vi "AtSpectrograph_logEvent_STRING.vi"(8 "error in (no error)":errorcluster, 11 "logevent_STRING_Ctl":T1) -> (0 "error out":errorcluster, 2 "function return":i32, 3 "logevent_STRING_Ctl out":T1)   [LabVIEW 2016, in "SALLV_AtSpectrograph.lvlib"]
doc: "int AtSpectrograph_shm_logEvent_STRINGLV(AtSpectrograph_logevent_STRINGLV *logevent_STRING_Ctl );"
uses:
  SALLV_AtSpectrograph.lvlib
  DataTypes/logevent_STRING.ctl
  SALLV_AtSpectrograph.so
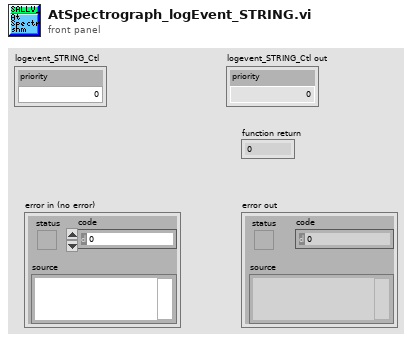
[diagram p1: front panel]
types:
  T1 = typedef "SALLV_AtSpectrograph.lvlib/logevent_STRING.ctl" = cluster{"priority":i32}
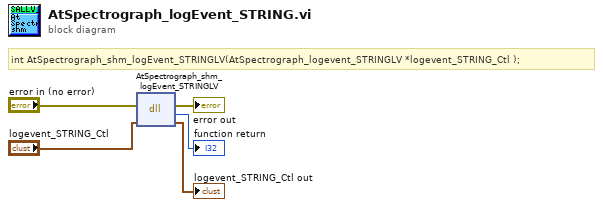
[diagram p0: block diagram]
diagram:
  # "int AtSpectrograph_shm_logEvent_STRINGLV(AtSpectrograph_logevent_STRINGLV *logevent_STRING_Ctl );"
  n1 = dll-call lib="home/harini/tcs/temp/SALLV_AtSpectrograph/SALLV_AtSpectrograph.*" fn="AtSpectrograph_shm_logEvent_STRINGLV"(error in="error in (no error)", "logevent_STRING_Ctl"="logevent_STRING_Ctl") -> (error out=→"error out":errorcluster, →"function return":i32, "logevent_STRING_Ctl"=→"logevent_STRING_Ctl out":T1)  [unwired: 2 in, 1 out]
